vi "End Sound.vi"   [LabVIEW 2020]
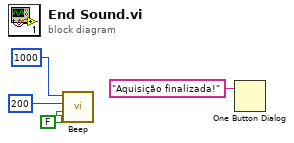
[diagram p0: block diagram]
diagram:
  n1 = call <vilib>:"Beep.vi"("use system alert? (T)"=FALSE, "duration (msec)"=u32 200, "frequency (Hz)"=u32 1000) -> ()  [unwired: 9 in]
  n2 = One Button Dialog(message="Aquisição finalizada!") -> ()  [unwired: 1 in, 1 out]
